vi "zad7.vi"(8 "error in (no error)":errorcluster, 9 "b 3":dbl, 10 "a":dbl, 11 "n":dbl) -> (1 "error out":errorcluster, 2 "f(X)":dbl[](array[numeric]))   [LabVIEW 2017]
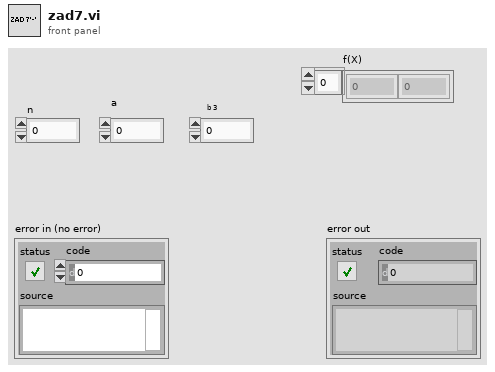
[diagram p1: front panel]
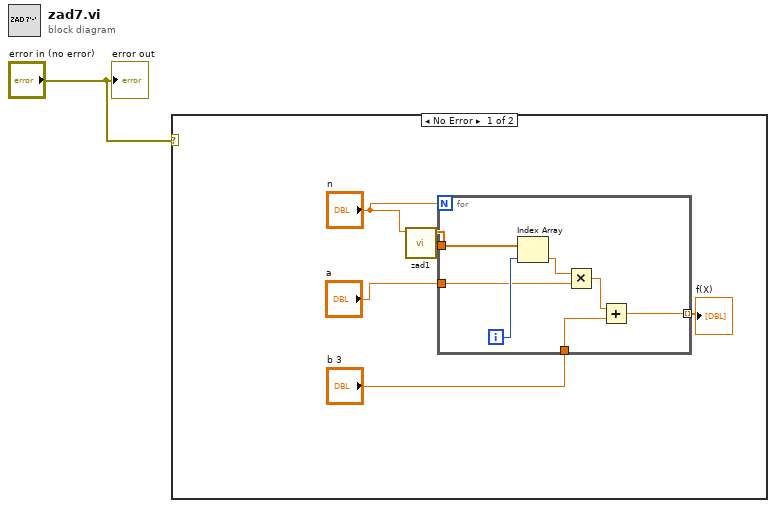
[diagram p0: block diagram]
diagram:
  n1 = case shown="No Error" "error in (no error)" {
    frame No Error {
      n2 = call "zad1.vi"("Numeric"="n") -> ("Array"=w5:dbl[])  [unwired: 9 in, 1 out]
      n3 = for {
        N: "n" -> [_]
        tunnel: w5 -> [w13]
        tunnel: "b 3" -> [w9]
        tunnel: [w8] -> w3 mode=indexing
        tunnel: "a" -> [w7]
        i -> [w12]
        n4 = Index Array(array=w13, index=w12) -> (element=w11:dbl)
        n5 = Multiply(x=w11, y=w7) -> (x*y=w10:dbl)
        n6 = Add(x=w10, y=w9) -> (x+y=w8:dbl)
      }
      "f(X)" <- w3
    }
    frame Error {
    }
  }
  "error out" <- "error in (no error)"
